vi "Dialog Core.vi"(6 "Variant in":variant, 7 "Shift Pressed?":bool, 8 "error in (no error)":errorcluster, 10 "QD Combo Box Ref":refnum<vi>, 11 "QD Launch VI Ref":refnum<vi>) -> (0 "error out":errorcluster, 4 "Variant out":variant)   [LabVIEW 2015, in "ScriptDialog.lvclass"]
uses:
  ScriptDialog.lvclass
  _Database/Ancestor/DatabaseAPI.lvclass
  Type Definitiions/Dialog Main ctls and VI ref.ctl
  ScriptDialog.lvclass/ScriptDialog.ctl
  System/Implements/SystemDialogConfiguration/ScriptsDialogConfiguration.lvclass
  <vilib>/addons/database/Auxilliary.llb/DB Tools Column Info.ctl
  <vilib>/addons/database/Auxilliary.llb/DB Tools DataTypes.ctl
  _Database/Implements/ScriptDatabase.lvclass
  _Database/Implements/ScriptDatabase.lvclass/ScriptDatabase.ctl
  <vilib>/Utility/error.llb/Error Cluster From Error Code.vi
  <vilib>/ErrorRing/Error Ring.xnode
  <vilib>/addons/database/NI_Database_API.lvlib
  System/UIConfiguration/UIConfiguration.lvclass
panel:
  in  "Search Contents":string
  in  "EchoQDFunction":bool
  in  "Search Result":i32(listbox)
  in  "Up":bool
  in  "Down":bool
  in  "Tools":cluster{"Configure":bool, "Help":bool}
  out "ToolLauncher out":refnum<class "ScriptDialog.lvclass">
  in  "Dialog":refnum<class "ScriptDialog.lvclass">
  in  "Stop":bool
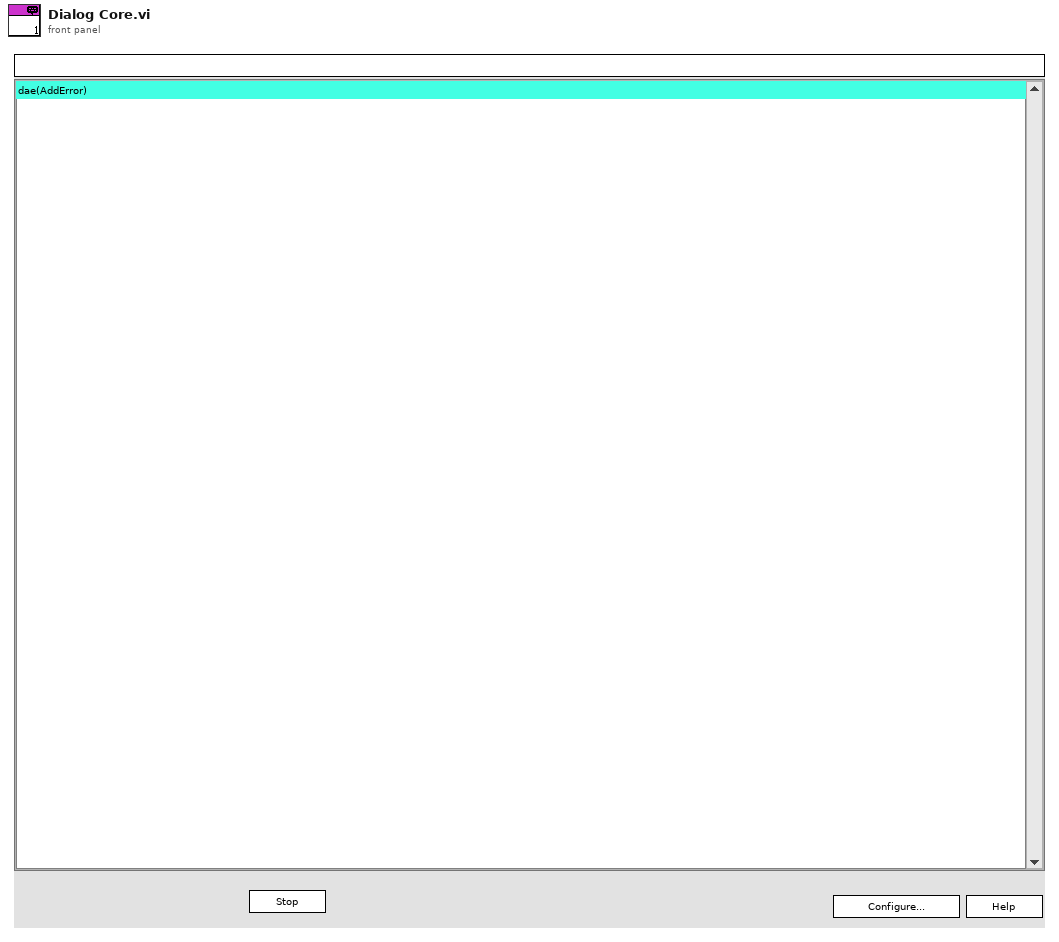
[diagram p1: front panel]
types:
  T1 = typedef "ScriptDialog.lvclass/Dialog Main ctls and VI ref.ctl" = cluster{"Search Results":refnum<vi>, "Search Contents":refnum<vi>, "Stop":refnum<vi>, "Help":refnum<vi>, "Configure":refnum<vi>, "Tools ":refnum<vi>, "Pane 2":refnum<vi>, "Splitter 2":refnum<vi>, "This VI":refnum<vi>}
  T2 = typedef "NI_Database_API.lvlib/DB Tools Column Info.ctl" = cluster{"column name":string, "data type":T3, "size":i32, "allow null?":bool}
  T3 = typedef "NI_Database_API.lvlib/DB Tools DataTypes.ctl" = enum16{"String", "Long (I32)", "Single (SGL)", "Double (DBL)", "Date/Time", "Binary"}
  T4 = typedef "eventvkey.ctl" = enum16{"ASCII", "Enter", "Return", "Shift", "Ctrl", "Alt", "Cmd", "Opt", "Caps", "NumLock", "Clear", "Break", "Up", "Down", "Left", "Right", "Insert", "Delete", "Home", "End", "PageUp", "PageDown", "Escape", "Help", "Pause", "ScrollLock", "F1", "F2", "F3", "F4", "F5", "F6", "F7", "F8", "F9", "F10", "F11", "F12", "F13", "F14", "F15", "F16", "F17", "F18", "F19", "F20", "F21", "F22", "F23", "F24", "Play", "VolumeUp", "VolumeDown", "Mute", "Two Byte Char"}
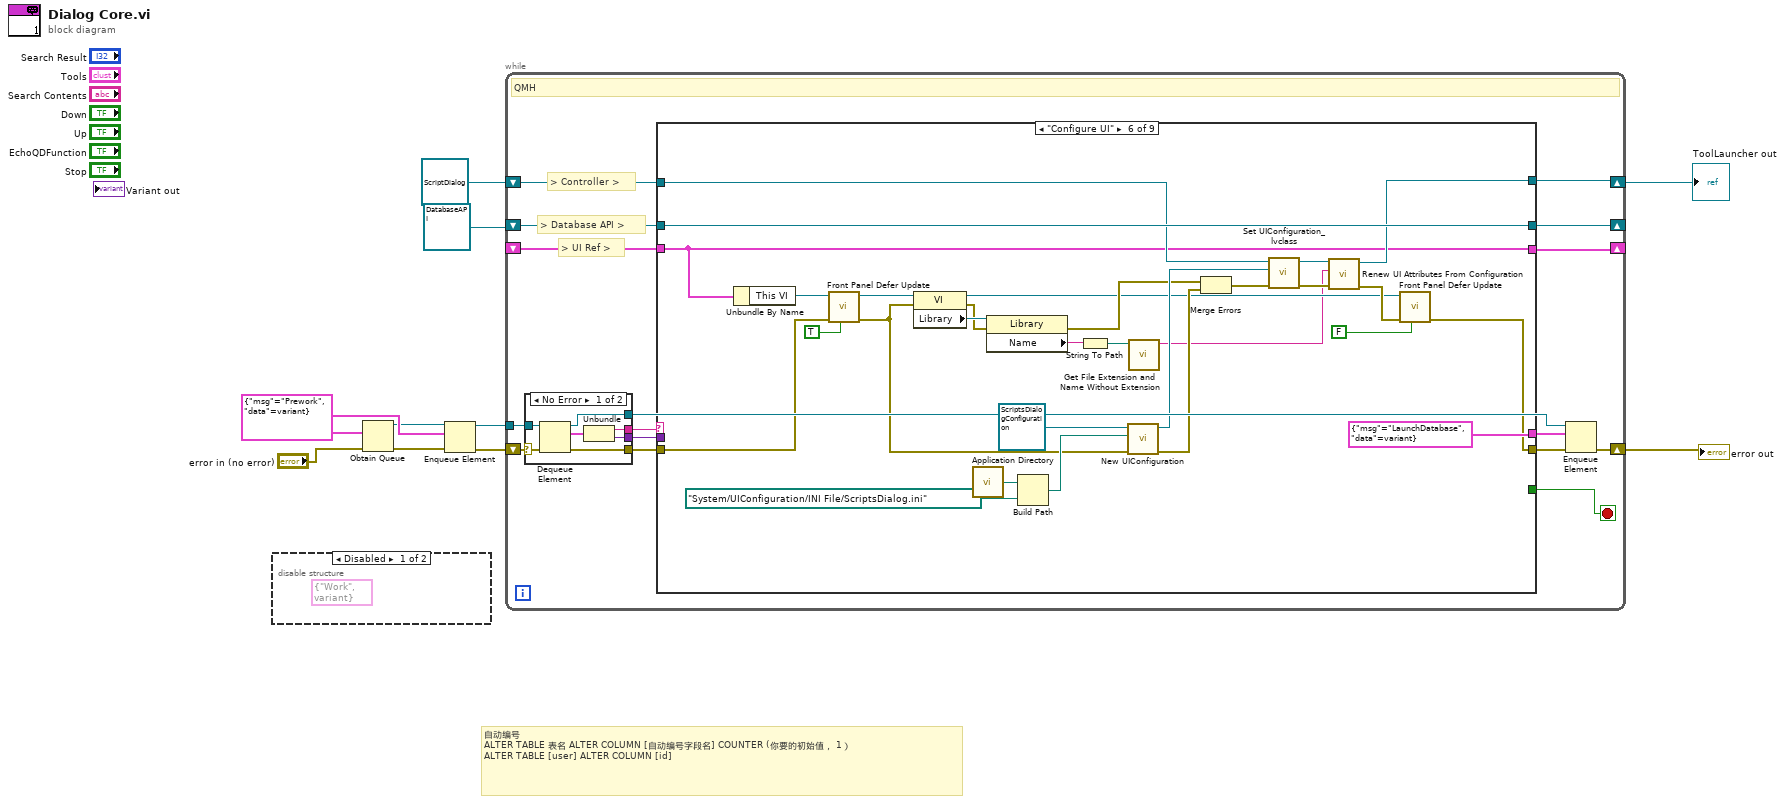
[diagram p0: block diagram]
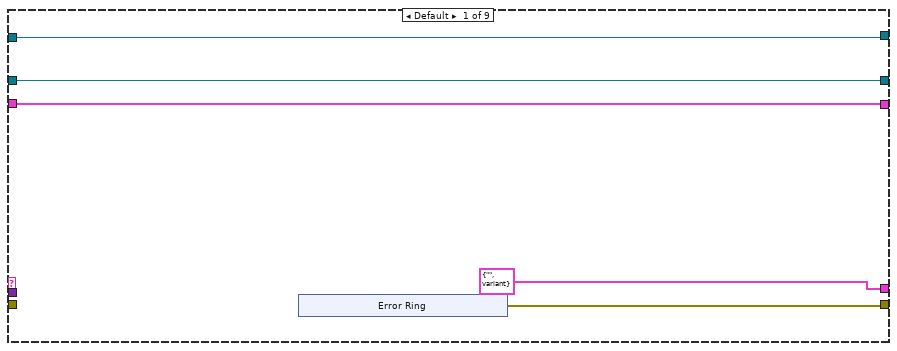
[diagram p3: hidden frame]
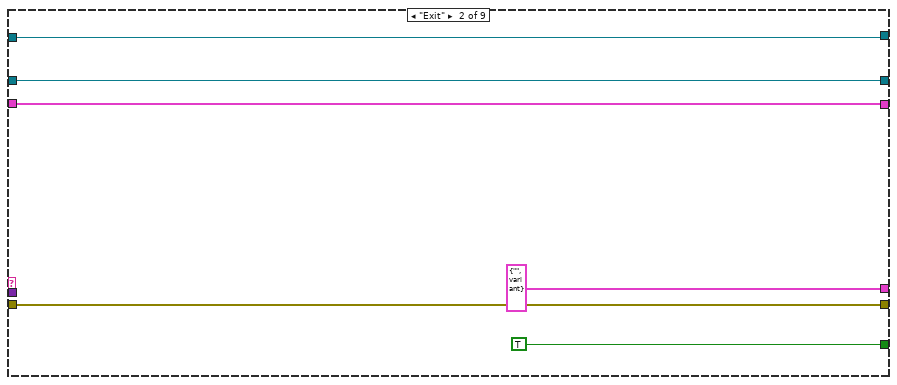
[diagram p4: hidden frame]
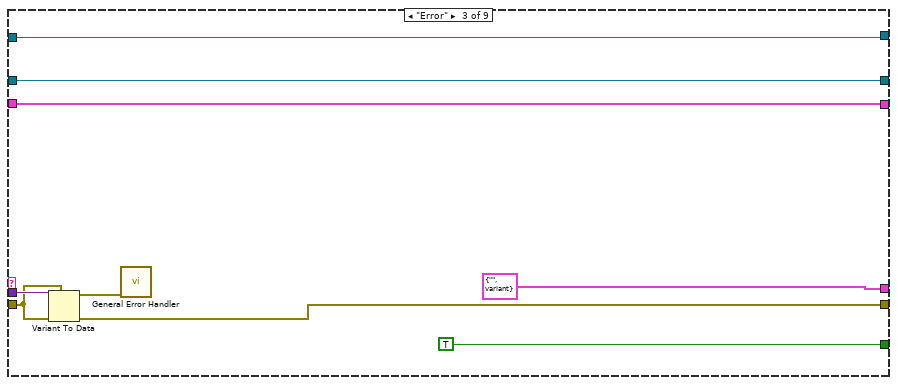
[diagram p5: hidden frame]
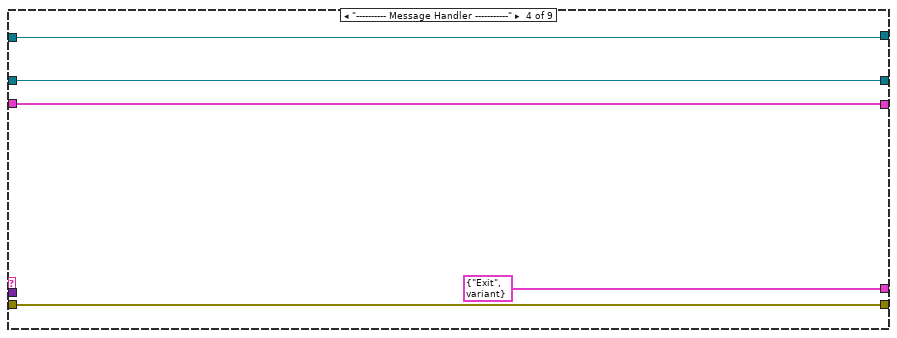
[diagram p6: hidden frame]
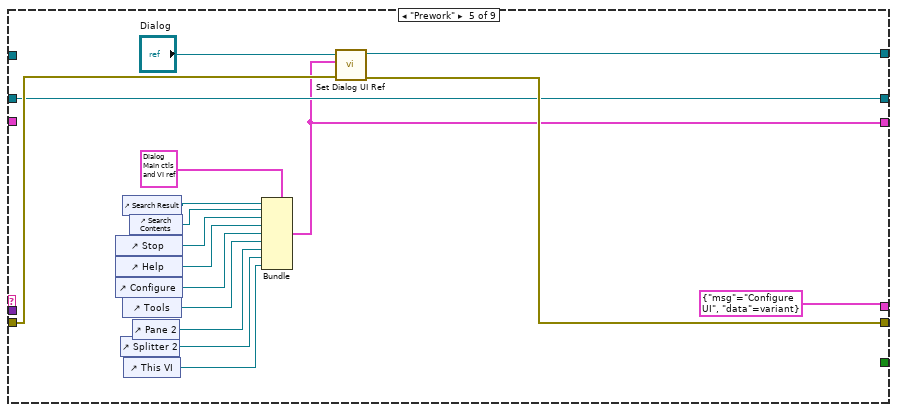
[diagram p7: hidden frame]
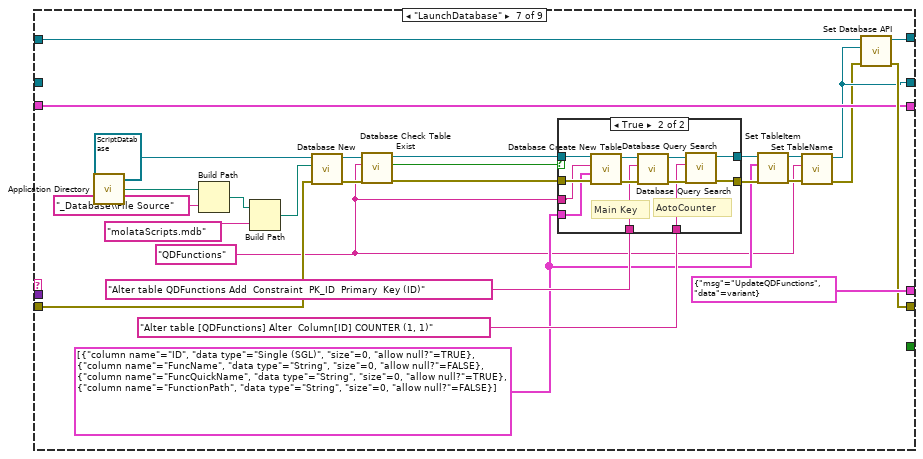
[diagram p8: hidden frame]
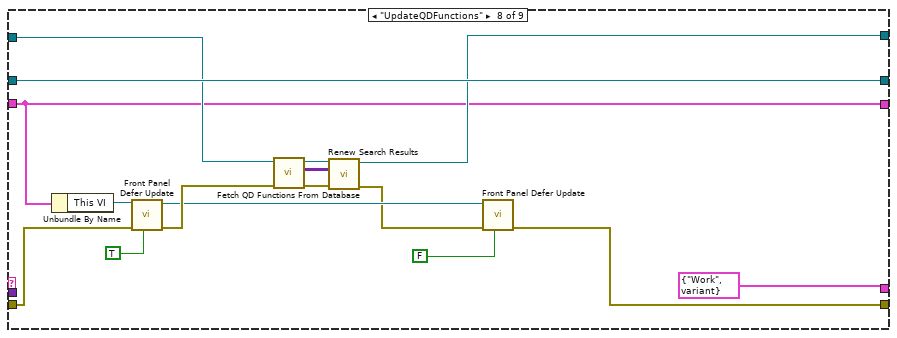
[diagram p10: hidden frame]
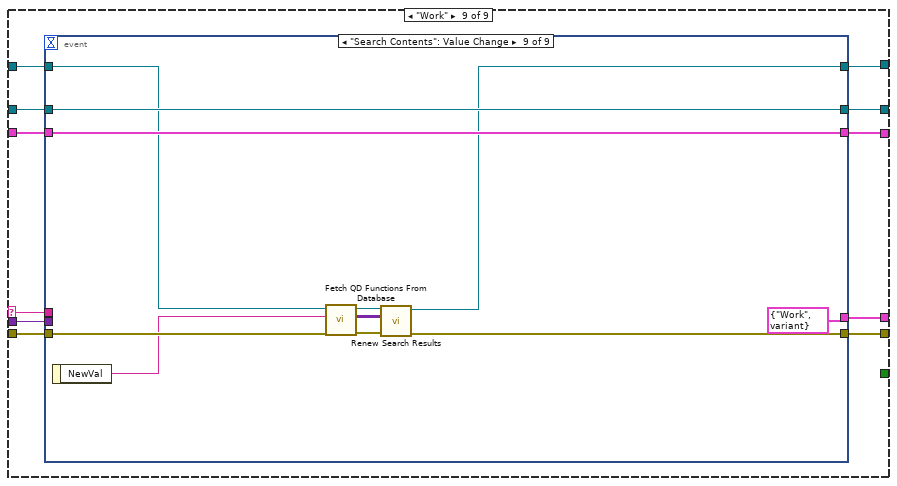
[diagram p11: hidden frame]
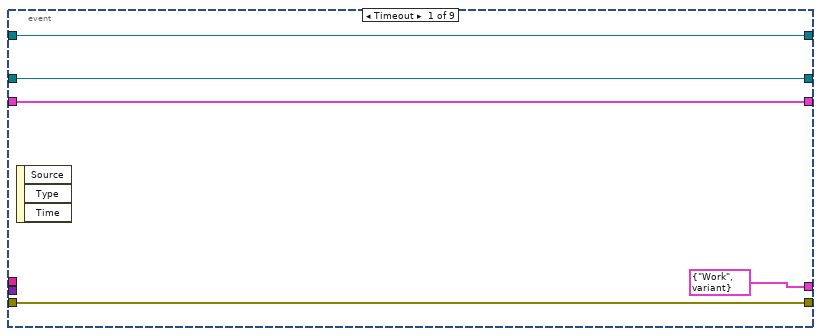
[diagram p12: hidden frame]
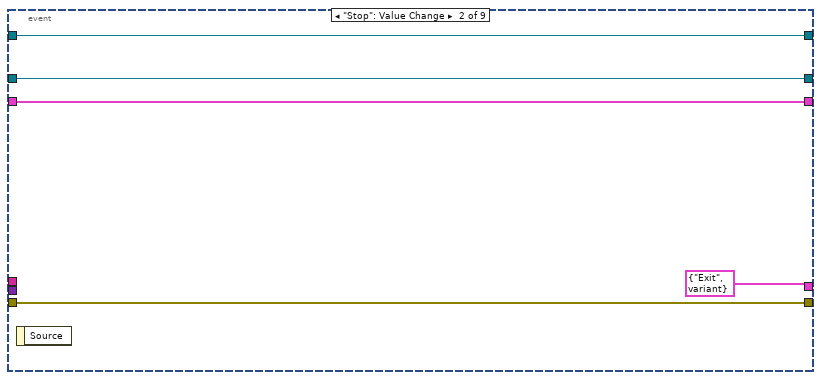
[diagram p13: hidden frame]
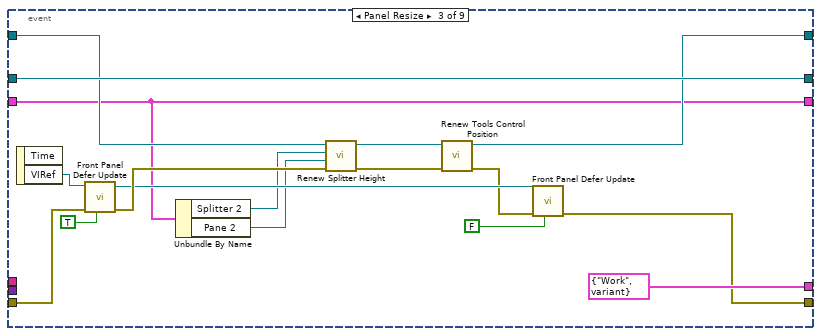
[diagram p14: hidden frame]
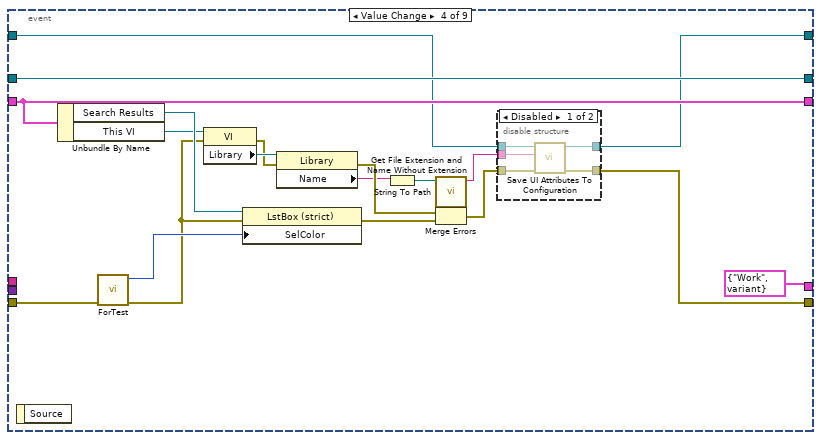
[diagram p15: hidden frame]
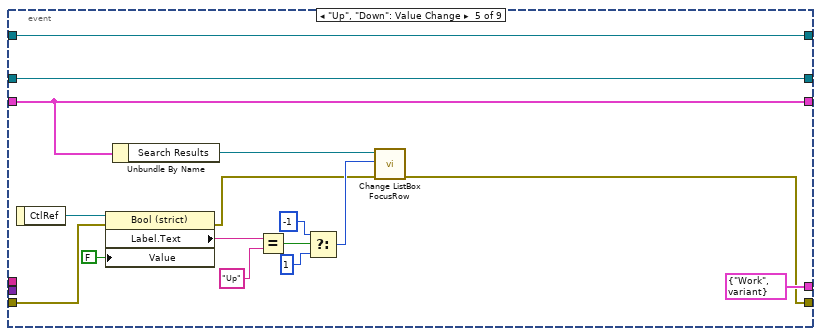
[diagram p17: hidden frame]
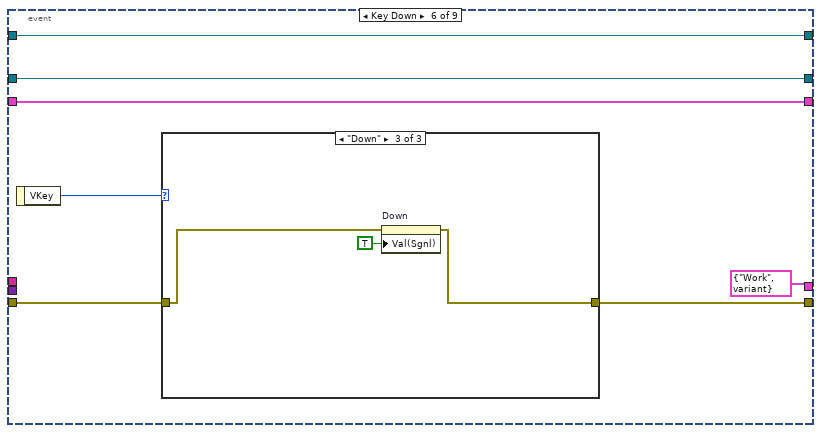
[diagram p18: hidden frame]
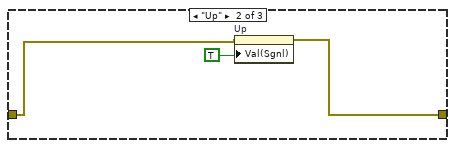
[diagram p20: hidden frame]
diagram:
  w8 = cluster{"msg":string, "data":variant} {"msg"="Prework", "data"=variant}
  # "自动编号\nALTER TABLE 表名 ALTER COLUMN [自动编号字段名] COUNTER (你要的初始值， 1）\nALTER TABLE [user] ALTER COLUMN [id]"
  n1 = disable-structure shown="Disabled" {
    frame Disabled {
      (unwired) cluster{"msg":string, "data":variant} {"msg"="Work", "data"=variant}
    }
    frame Enabled {
    }
  }
  n2 = Obtain Queue(element data type=w8, error in (no error)="error in (no error)") -> (queue out=w6:refnum<queue>, error out=w7:errorcluster)  [unwired: 3 in, 1 out]
  n3 = Enqueue Element(queue=w6, element=w8, error in (no error)=w7) -> (queue out=w9:refnum<queue>, error out=w10:errorcluster)  [unwired: 1 in, 1 out]
  n4 = while {
    tunnel: w9 -> [w25]
    shift-right: [w20] -> w1
    shift-left: w10 -> [w26]
    shift-right: [w15] -> w3
    shift-left: refnum<class "ScriptDialog.lvclass"> refnum ("ScriptDialog out") -> [w16]
    shift-right: [w14] -> _
    shift-left: refnum<class "DatabaseAPI.lvclass"> refnum ("object out") -> [w13]
    shift-right: [w12] -> _
    shift-left: _ -> [w11]
    stop <- w17 stop-if-true
    # "> UI Ref >"
    # "> Database API >"
    # "> Controller >"
    # "QMH"
    n5 = case shown="No Error" w26 {
      selector: w26 -> [w294 w298]
      tunnel: w25 -> [w295 w296]
      tunnel: [w293 _] -> w24
      tunnel: [w291 "Error" ("msg")] -> w23
      tunnel: [w290 w298] -> w22
      tunnel: [w289 w296] -> w19
      frame No Error {
        n6 = Dequeue Element(queue=w295, error in (no error)=w294) -> (queue out=w289:refnum<queue>, element=w292:cluster{"msg":string, "data":variant}, error out=w293:errorcluster)  [unwired: 1 in, 1 out]
        n7 = Unbundle(w292) -> ("msg"=w291:string, "data"=w290:variant)
      }
      frame Error {
      }
    }
    n8 = case shown="\"Configure UI\"" w23 {
      selector: w23 -> [_ _ _ _ _ _ _ _ w168]
      tunnel: w24 -> [_ w42 w50 w56 w67 w89 w124 w150 w170]
      tunnel: w22 -> [_ _ w51 _ _ _ _ _ w169]
      tunnel: [w31 w42 w48 w56 w66 w86 w121 w146 w167] -> w21
      tunnel: [cluster{"msg":string, "data":variant} {"msg"="", "data"=variant} cluster{"msg":string, "data":variant} {"msg"="", "data"=variant} cluster{"msg":string, "data":variant} {"msg"="", "data"=variant} cluster{"msg":string, "data":variant} {"msg"="Exit", "data"=variant} cluster{"msg":string, "data":variant} {"msg"="Configure UI", "data"=variant} cluster{"msg":string, "data":variant} {"msg"="LaunchDatabase", "data"=variant} cluster{"msg":string, "data":variant} {"msg"="UpdateQDFunctions", "data"=variant} cluster{"msg":string, "data":variant} {"msg"="Work", "data"=variant} w166] -> w18
      tunnel: [_ TRUE TRUE _ _ _ _ _ _] -> w17
      tunnel: w16 -> [w28 w38 w44 w53 _ w96 w122 w157 w165]
      tunnel: [w28 w38 w44 w53 w65 w92 w120 w153 w163] -> w15
      tunnel: [w29 w39 w45 w54 w63 w102 w106 w159 w162] -> w14
      tunnel: w13 -> [w29 w39 w45 w54 w63 w102 _ w159 w164]
      tunnel: [w27 w37 w43 w52 w62 w91 w119 w152 w160] -> w12
      tunnel: w11 -> [w27 w37 w43 w52 _ w91 w119 w152 w161]
      frame Default {
        n9 = xnode "Error Ring"() -> ("error out"=w31:errorcluster)
      }
      frame "Exit" {
      }
      frame "Error" {
        n10 = Variant To Data(error in=w50, type=w50, Variant=w51) -> (data=w49:errorcluster, error out=w48:errorcluster)
        n11 = call <vilib>:"General Error Handler.vi"("error in (no error)"=w49) -> ()  [unwired: 10 in, 5 out]
      }
      frame "---------- Message Handler -----------" {
      }
      frame "Prework" {
        n12 = control-ref of="Stop"() -> (w71:refnum<vi>)
        n13 = control-ref of="Help"() -> (w70:refnum<vi>)
        n14 = control-ref of="Configure"() -> (w69:refnum<vi>)
        n15 = control-ref of="Splitter 2"() -> (w59:refnum<vi>)
        n16 = control-ref of="Search Result"() -> (w57:refnum<vi>)
        n17 = control-ref of="Tools"() -> (w61:refnum<vi>)
        n18 = control-ref of="This VI"() -> (w58:refnum<vi>)
        n19 = control-ref of="Search Contents"() -> (w72:refnum<vi>)
        n20 = control-ref of="Pane 2"() -> (w60:refnum<vi>)
        n21 = Bundle(cluster=T1 {"Search Results"=refnum, "Search Contents"=refnum, "Stop"=refnum, "Help"=refnum, "Configure"=refnum, "Tools "=refnum, "Pane 2"=refnum, "Splitter 2"=refnum, "This VI"=refnum}, "Search Results"=w57, "Search Contents"=w72, "Stop"=w71, "Help"=w70, "Configure"=w69, "Tools"=w61, "Pane 2"=w60, "Splitter 2"=w59, "This VI"=w58) -> (w62:T1)
        n22 = call "Set Dialog UI Ref.vi"("error in (no error)"=w67, "Main ctls and VI ref"=w62, "ScriptDialog in"="Dialog") -> ("error out"=w66:errorcluster, "ScriptDialog out"=w65:refnum<class "ScriptDialog.lvclass">)  [unwired: 7 in]
      }
      frame "Configure UI" {
        n23 = Unbundle By Name(w91) -> ("This VI"=w90:refnum<vi>)
        n24 = call <userlib>:"Front Panel Defer Update.vi"("Defer Panel Updates(False)"=TRUE, "error in (no error)"=w89, "This VI"=w90) -> ("error out"=w81:errorcluster, "This VI Out"=w82:refnum<vi>)  [unwired: 7 in]
        n25 = property class="VI"(reference=w82, error in=w81) -> (reference out=w77:refnum<vi>, error out=w83:errorcluster, "Library"=w84:refnum<vi>)
        n26 = call <vilib>:"Application Directory.vi"() -> ("Application Directory"=w100:path)
        n27 = property class="Library"(reference=w84, error in=w83) -> (error out=w80:errorcluster, "Name"=w75:string)  [unwired: 1 out]
        n28 = Build Path(base path=w100, name or relative path=path "System/UIConfiguration/INI File/ScriptsDialog.ini" ("Path")) -> (appended path=w98:path)
        n29 = String To Path(string=w75) -> (path=w76:path)
        n30 = call "New UIConfiguration.vi"("error in (no error)"=w81, "Ini"=w98, "UIConfiguration in"=refnum<class "ScriptsDialogConfiguration.lvclass"> refnum ("ScriptsDialogConfiguration")) -> ("error out"=w79:errorcluster, "UIConfiguration out"=w95:refnum<class "ScriptsDialogConfiguration.lvclass">)  [unwired: 7 in]
        n31 = call <userlib>:"Get File Extension and Name Without Extension.vi"("file"=w76) -> ("filename without extension"=w74:string)  [unwired: 9 in, 1 out]
        n32 = Merge Errors(w80, w79) -> (w78:errorcluster)
        n33 = call "Set UIConfiguration_lvclass.vi"("error in (no error)"=w78, "UIConfiguration.lvclass"=w95, "ScriptDialog in"=w96) -> ("error out"=w93:errorcluster, "ScriptDialog out"=w94:refnum<class "ScriptDialog.lvclass">)  [unwired: 7 in]
        n34 = call "Renew UI Attributes From Configuration.vi"("error in (no error)"=w93, "section"=w74, "ScriptDialog in"=w94) -> ("error out"=w87:errorcluster, "ScriptDialog out"=w92:refnum<class "ScriptDialog.lvclass">)  [unwired: 7 in]
        n35 = call <userlib>:"Front Panel Defer Update.vi"("Defer Panel Updates(False)"=FALSE, "error in (no error)"=w87, "This VI"=w77) -> ("error out"=w86:errorcluster)  [unwired: 7 in, 1 out]
      }
      frame "LaunchDatabase" {
        w104 = T2[] [{"column name"="ID", "data type"=enum."Single (SGL)", "size"=0, "allow null?"=TRUE}, {"column name"="FuncName", "data type"=enum."String", "size"=0, "allow null?"=FALSE}, {"column name"="FuncQuickName", "data type"=enum."String", "size"=0, "allow null?"=TRUE}, {"column name"="FunctionPath", "data type"=enum."String", "size"=0, "allow null?"=FALSE}] ("column information")
        w103 = "QDFunctions" ("Table")
        n36 = call <vilib>:"Application Directory.vi"() -> ("Application Directory"=w129:path)
        n37 = Build Path(base path=w129, name or relative path="_Database\\File Source") -> (appended path=w127:path)
        n38 = Build Path(base path=w127, name or relative path="molataScripts.mdb") -> (appended path=w125:path)
        n39 = call "Database New.vi"("error in (no error)"=w124, "Database File Path"=w125, "object in"=refnum<class "ScriptDatabase.lvclass"> refnum ("ScriptDatabase")) -> ("error out"=w117:errorcluster, "object out"=w118:refnum<class "ScriptDatabase.lvclass">)  [unwired: 7 in]
        n40 = call "Database Check Table Exist.vi"("error in (no error)"=w117, "Table Name(\"\")"=w103, "Database in"=w118) -> ("error out"=w115:errorcluster, "Exit?(True)"=w114:bool, "Database out"=w116:refnum<class "ScriptDatabase.lvclass">)  [unwired: 6 in]
        n41 = case shown="True" w114 {
          tunnel: w116 -> [w131 w143]
          tunnel: w115 -> [w130 w142]
          tunnel: w103 -> [_ w137]
          tunnel: w104 -> [_ w139]
          tunnel: [w131 w133] -> w108
          tunnel: [w130 w132] -> w107
          tunnel: "Alter table QDFunctions Add  Constraint  PK_ID  Primary  Key (ID)" ("SQL query") -> [_ w138]
          tunnel: "Alter table [QDFunctions] Alter  Column[ID] COUNTER (1, 1)" ("SQL query") -> [_ w134]
          frame False {
          }
          frame True {
            # "AotoCounter"
            # "Main Key"
            n42 = call "Database Create New Table.vi"("error in (no error)"=w142, "column information"=w139, "table"=w137, "Database in"=w143) -> ("error out"=w140:errorcluster, "Database out"=w141:refnum<class "ScriptDatabase.lvclass">)  [unwired: 6 in]
            n43 = call "Database Query Search.vi"("error in (no error)"=w140, "SQL query"=w138, "Database in"=w141) -> ("error out"=w136:errorcluster, "Database out"=w135:refnum<class "ScriptDatabase.lvclass">)  [unwired: 7 in]
            n44 = call "Database Query Search.vi"("error in (no error)"=w136, "SQL query"=w134, "Database in"=w135) -> ("error out"=w132:errorcluster, "Database out"=w133:refnum<class "ScriptDatabase.lvclass">)  [unwired: 7 in]
          }
        }
        n45 = call "Set TableItem.vi"("error in (no error)"=w107, "TableItem"=w104, "ScriptDatabase in"=w108) -> ("error out"=w109:errorcluster, "ScriptDatabase out"=w110:refnum<class "ScriptDatabase.lvclass">)  [unwired: 7 in]
        n46 = call "Set TableName.vi"("error in (no error)"=w109, "TableName"=w103, "ScriptDatabase in"=w110) -> ("error out"=w105:errorcluster, "ScriptDatabase out"=w106:refnum<class "ScriptDatabase.lvclass">)  [unwired: 7 in]
        n47 = call "Set Database API.vi"("error in (no error)"=w105, "ScriptDatabase"=w106, "ScriptDialog in"=w122) -> ("error out"=w121:errorcluster, "ScriptDialog out"=w120:refnum<class "ScriptDialog.lvclass">)  [unwired: 7 in]
      }
      frame "UpdateQDFunctions" {
        n48 = Unbundle By Name(w152) -> ("This VI"=w151:refnum<vi>)
        n49 = call <userlib>:"Front Panel Defer Update.vi"("Defer Panel Updates(False)"=TRUE, "error in (no error)"=w150, "This VI"=w151) -> ("error out"=w149:errorcluster, "This VI Out"=w148:refnum<vi>)  [unwired: 7 in]
        n50 = call "Fetch QD Functions From Database.vi"("error in (no error)"=w149, "ToolLauncher in"=w157) -> ("error out"=w155:errorcluster, "QDFunctionsData"=w154:variant[][], "ToolLauncher out"=w156:refnum<class "ScriptDialog.lvclass">)  [unwired: 7 in]
        n51 = call "Renew Search Results.vi"("error in (no error)"=w155, "QDFunctionsData"=w154, "ScriptDialog in"=w156) -> ("error out"=w147:errorcluster, "ScriptDialog out"=w153:refnum<class "ScriptDialog.lvclass">)  [unwired: 7 in]
        n52 = call <userlib>:"Front Panel Defer Update.vi"("Defer Panel Updates(False)"=FALSE, "error in (no error)"=w147, "This VI"=w148) -> ("error out"=w146:errorcluster)  [unwired: 7 in, 1 out]
      }
      frame "Work" {
        n53 = event shown="[8] \"Search Contents\": Value Change" {
          selector: _ -> [_ _ _ _ _ _ _ _ _]
          dyn-events: _ -> [_ _ _ _ _ _ _ _ _]
          timeout: _ -> [_ _ _ _ _ _ _ _ _]
          tunnel: w170 -> [w175 w180 w191 w215 w233 w241 w255 w274 w283]
          tunnel: w169 -> [_ _ _ _ _ _ _ _ _]
          tunnel: w168 -> [_ _ _ _ _ _ _ _ _]
          tunnel: [w175 w180 w185 w209 w225 w240 w259 w272 w279] -> w167
          tunnel: [cluster{"msg":string, "data":variant} {"msg"="Work", "data"=variant} cluster{"msg":string, "data":variant} {"msg"="Exit", "data"=variant} cluster{"msg":string, "data":variant} {"msg"="Work", "data"=variant} cluster{"msg":string, "data":variant} {"msg"="Work", "data"=variant} cluster{"msg":string, "data":variant} {"msg"="Work", "data"=variant} cluster{"msg":string, "data":variant} {"msg"="Work", "data"=variant} cluster{"msg":string, "data":variant} {"msg"="Work", "data"=variant} cluster{"msg":string, "data":variant} {"msg"="Work", "data"=variant} cluster{"msg":string, "data":variant} {"msg"="Work", "data"=variant}] -> w166
          tunnel: w165 -> [w173 w178 w193 w211 w239 w246 w267 w277 w282]
          tunnel: w164 -> [w172 w177 w196 w216 w238 w245 w270 w276 w288]
          tunnel: [w173 w178 w189 w210 w239 w246 w260 w277 w280] -> w163
          tunnel: [w172 w177 w196 w216 w238 w245 w270 w276 w288] -> w162
          tunnel: w161 -> [w171 w176 w184 w214 w237 w244 w269 w275 w287]
          tunnel: [w171 w176 w184 w214 w237 w244 w269 w275 w287] -> w160
          event Timeout {
            n54 = event-data() -> ()  [unwired: 1 in, 3 out]
          }
          event "Stop": Value Change {
            n55 = event-data() -> ()  [unwired: 1 in, 1 out]
          }
          event Panel Resize {
            n56 = event-data() -> ("VIRef"=w192:refnum<vi>)  [unwired: 1 in, 1 out]
            n57 = call <userlib>:"Front Panel Defer Update.vi"("Defer Panel Updates(False)"=TRUE, "error in (no error)"=w191, "This VI"=w192) -> ("error out"=w190:errorcluster, "This VI Out"=w187:refnum<vi>)  [unwired: 7 in]
            n58 = Unbundle By Name(w184) -> ("Splitter 2"=w183:refnum<vi>, "Pane 2"=w182:refnum<vi>)
            n59 = call "Renew Splitter Height.vi"("error in (no error)"=w190, "Pane Ref"=w182, "Splitter Ref"=w183, "ScriptDialog.lvclass"=w193) -> ("error out"=w194:errorcluster, "ScriptDialog.lvclass Out"=w195:refnum<class "ScriptDialog.lvclass">)  [unwired: 6 in]
            n60 = call "Renew Tools Control Position.vi"("error in (no error)"=w194, "ScriptDialog"=w195) -> ("error out"=w186:errorcluster, "ScriptDialog  Out"=w189:refnum<class "ScriptDialog.lvclass">)  [unwired: 8 in]
            n61 = call <userlib>:"Front Panel Defer Update.vi"("Defer Panel Updates(False)"=FALSE, "error in (no error)"=w186, "This VI"=w187) -> ("error out"=w185:errorcluster)  [unwired: 7 in, 1 out]
          }
          event "Tools.Configure": Value Change {
            n62 = event-data() -> ()  [unwired: 1 in, 1 out]
            n63 = Unbundle By Name(w214) -> ("Search Results"=w213:refnum<vi>, "This VI"=w207:refnum<vi>)
            n64 = call "ForTest.vi"("error in (no error)"=w215) -> ("error out"=w206:errorcluster, "Color Out"=w212:u32)  [unwired: 9 in]
            n65 = property class="VI"(reference=w207, error in=w206) -> (error out=w202:errorcluster, "Library"=w203:refnum<vi>)  [unwired: 1 out]
            n66 = property class="LstBox (strict)"(reference=w213, error in=w206, "SelColor"=w212) -> (error out=w205:errorcluster)  [unwired: 1 out]
            n67 = property class="Library"(reference=w203, error in=w202) -> (error out=w201:errorcluster, "Name"=w200:string)  [unwired: 1 out]
            n68 = String To Path(string=w200) -> (path=w199:path)
            n69 = call <userlib>:"Get File Extension and Name Without Extension.vi"("file"=w199) -> ("filename without extension"=w198:string)  [unwired: 9 in, 1 out]
            n70 = Merge Errors(w201, w205) -> (w204:errorcluster)
            n71 = disable-structure shown="Disabled" {
              disable-tunnel: w211 -> [w221 w223]
              disable-tunnel: [w220 w223] -> w210
              disable-tunnel: [w219 w222] -> w209
              disable-tunnel: w198 -> [w218 _]
              disable-tunnel: w204 -> [w217 w222]
              frame Disabled {
                n72 = call "Save UI Attributes To Configuration.vi"("error in (no error)"=w217, "Selection Name"=w218, "ScriptDialog in"=w221) -> ("error out"=w219:errorcluster, "ScriptDialog out"=w220:refnum<class "ScriptDialog.lvclass">)  [unwired: 7 in]
              }
              frame Enabled {
              }
            }
          }
          event "Up", "Down": Value Change {
            n73 = event-data() -> ("CtlRef"=w234:refnum<vi>)  [unwired: 1 in]
            n74 = property class="Bool (strict)"(reference=w234, error in=w233, "Value"=FALSE) -> (error out=w226:errorcluster, "Label.Text"=w232:string)  [unwired: 1 out]
            n75 = Unbundle By Name(w237) -> ("Search Results"=w235:refnum<vi>)
            n76 = Equal?(x=w232, y="Up") -> (x = y?=w230:bool)
            n77 = Select(t=-1 ("Variation"), s=w230, f=1 ("Variation")) -> (s? t:f=w227:i32)
            n78 = call <userlib>:"Change ListBox FocusRow.vi"("error in (no error)"=w226, "Variation"=w227, "LstBox Refnum"=w235) -> ("error out"=w225:errorcluster)  [unwired: 7 in, 1 out]
          }
          event Key Down {
            n79 = event-data() -> ("VKey"=w242:T4)  [unwired: 1 in]
            n80 = case shown="\"Down\"" w242 {
              tunnel: w241 -> [w247 w250 w252]
              tunnel: [w247 w249 w251] -> w240
              frame Default {
              }
              frame "Up" {
                n81 = property on="Up" class="Bool (strict)"(error in=w250, "Val(Sgnl)"=TRUE ("Value (Signaling)")) -> (error out=w249:errorcluster)  [unwired: 1 in, 1 out]
              }
              frame "Down" {
                n82 = property on="Down" class="Bool (strict)"(error in=w252, "Val(Sgnl)"=TRUE ("Value (Signaling)")) -> (error out=w251:errorcluster)  [unwired: 1 in, 1 out]
              }
            }
          }
          event "EchoQDFunction": Value Change {
            n83 = event-data() -> ("CtlRef"=w257:refnum<vi>)  [unwired: 1 in]
            n84 = property class="Bool (strict)"(reference=w257, error in=w255, "Value"=FALSE) -> (error out=w254:errorcluster)  [unwired: 1 out]
            n85 = Unbundle By Name(w269) -> ("Search Results"=w268:refnum<vi>)
            n86 = call <userlib>:"Get Listbox FocusRow Text.vi"("error in (no error)"=w254, "LstBox Refnum"=w268) -> ("error out"=w265:errorcluster, "Selected Item"=w266:string)  [unwired: 6 in, 2 out]
            n87 = call "Echo Scripts.vi"("ToolLauncher in"=w267, "Shift Pressed?"="Shift Pressed?", "QD Launch VI Ref"="QD Launch VI Ref", "QD Combo Box Ref"="QD Combo Box Ref", "QDFunctions"=w266, "error in (no error)"=w265, "Variant in"="Variant in") -> ("ToolLauncher out"=w260:refnum<class "ScriptDialog.lvclass">, "error out"=w259:errorcluster)  [unwired: 7 in]
          }
          event "Search Result": Double Click {
            n88 = event-data() -> ()  [unwired: 1 in, 1 out]
            n89 = property on="EchoQDFunction" class="Bool (strict)"(error in=w274, "Val(Sgnl)"=TRUE ("Value (Signaling)")) -> (error out=w272:errorcluster)  [unwired: 1 in, 1 out]
          }
          event "Search Contents": Value Change {
            n90 = event-data() -> ("NewVal"=w281:string)  [unwired: 1 in]
            n91 = call "Fetch QD Functions From Database.vi"("error in (no error)"=w283, "Keyword(\"\")"=w281, "ToolLauncher in"=w282) -> ("error out"=w285:errorcluster, "QDFunctionsData"=w284:variant[][], "ToolLauncher out"=w286:refnum<class "ScriptDialog.lvclass">)  [unwired: 6 in]
            n92 = call "Renew Search Results.vi"("error in (no error)"=w285, "QDFunctionsData"=w284, "ScriptDialog in"=w286) -> ("error out"=w279:errorcluster, "ScriptDialog out"=w280:refnum<class "ScriptDialog.lvclass">)  [unwired: 7 in]
          }
        }
      }
    }
    n93 = Enqueue Element(queue=w19, element=w18, error in (no error)=w21) -> (error out=w20:errorcluster)  [unwired: 1 in, 2 out]
  }
  "ToolLauncher out" <- w3
  "error out" <- w1
